vi "Cal3-GetSetup.vi"(6 "Sampling speeds":T3={"Samples/ch"=600, "Sample Rate/ch (Hz)"=100.0} {"Sample Rate/ch (Hz)" min=0; "Samples/ch" min=0 step=1}, 7 "data mode":enum16{"Take new data point", "Refit Curve"}(ring), 9 "Fixed n":bool, 10 "Mode in":T2, 11 "Boolean in":bool) -> (1 "Sampling speeds Output":T1, 2 "Fixed n out":bool, 3 "Boolean out":bool)   [LabVIEW 2016]
uses:
  Anemometry Sub Vis/Calibration/Calib_mode.ctl
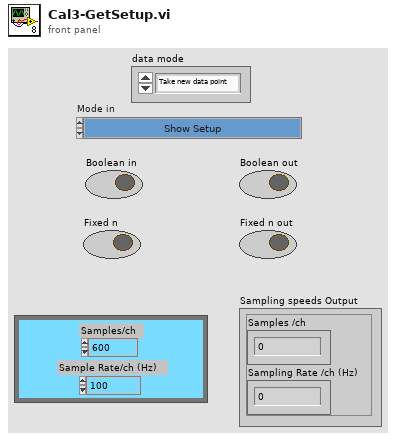
[diagram p1: front panel]
types:
  T1 = cluster{"Samples /ch":i32, "Sampling Rate /ch (Hz)":sgl}
  T2 = typedef "Calib_mode.ctl" = enum16{"Show Setup", "Take a New Calibration Point", "Refit Curve", "Setup Front Panel"}
  T3 = cluster{"Samples/ch":i32, "Sample Rate/ch (Hz)":sgl}
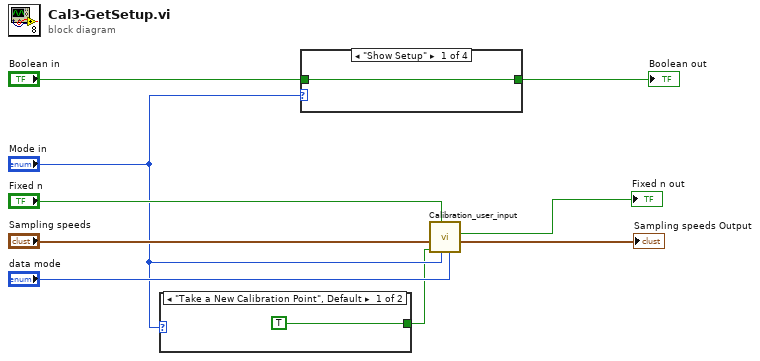
[diagram p0: block diagram]
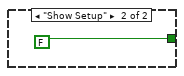
[diagram p2: hidden frame]
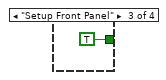
[diagram p4: hidden frame]
diagram:
  n1 = case shown="\"Take a New Calibration Point\", Default" "Mode in" {
    tunnel: [TRUE ("OK") FALSE ("OK")] -> w1
    frame "Take a New Calibration Point", Default {
    }
    frame "Show Setup" {
    }
  }
  n2 = case shown="\"Show Setup\"" "Mode in" {
    tunnel: [w12 w13 TRUE w15] -> w8
    tunnel: "Boolean in" -> [w12 w13 _ w15]
    frame "Show Setup" {
    }
    frame "Refit Curve" {
    }
    frame "Setup Front Panel" {
    }
    frame "Take a New Calibration Point" {
    }
  }
  "Boolean out" <- w8
  n3 = call "Calibration_user_input.vi"("data mode"="data mode", "Mode"="Mode in", "Fixed n"="Fixed n", "OK"=w1, "Sampling speeds"="Sampling speeds") -> ("Sampling speeds Output"=→"Sampling speeds Output":T1, "Fixed n out"=→"Fixed n out":bool)  [unwired: 2 in, 3 out]
